vi "Find New Visa.vi"(8 "error in (no error)":errorcluster caption="entrée d'erreur (pas d'erreur)", 11 "Fonction":enum16{"Lecture Liste", "Recherche Nouveau"}(ring)=enum."Recherche Nouveau") -> (0 "error out":errorcluster caption="sortie d'erreur", 1 "Com à Initialiser":string, 2 "Trouvé":bool, 3 "liste trouvée":string[](array[string]))   [LabVIEW 2020]
uses:
  <vilib>/Instr/_visa.llb/VISA Find Search Mode.ctl
  IHM/Variable globale.vi
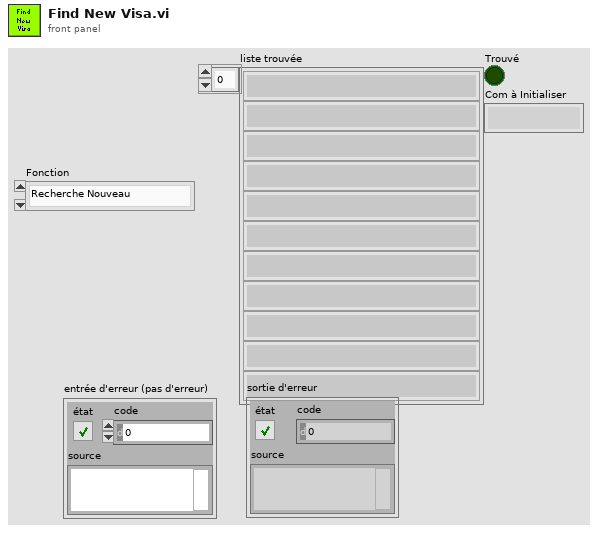
[diagram p1: front panel]
types:
  T1 = typedef "VISA Find Search Mode.ctl" = u32
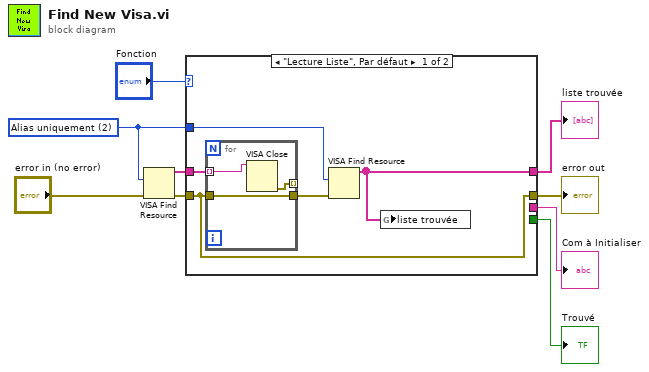
[diagram p0: block diagram]
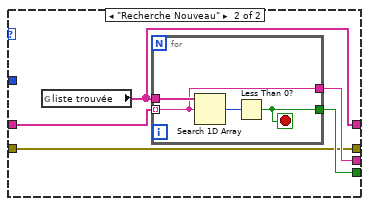
[diagram p2: hidden frame]
diagram:
  w1 = T1 2 items=["Noms canoniques uniquement"=0, "Alias uniquement"=2, "Inclure les alias correspondants"=3, "Inclure tous les alias"=4] ("Search Mode")
  n1 = VISA Find Resource(8:"error in (no error)", 10:w1) -> (0:w8:errorcluster, 3:w5:string[])  [unwired: 1 in, 1 out]
  n2 = case shown="\"Lecture Liste\", Par défaut" "Fonction" {
    tunnel: [w11 w18] -> w4
    tunnel: w5 -> [w12 w20]
    tunnel: [w14 w19] -> w2
    tunnel: w8 -> [w14 w19]
    tunnel: [_ w22] -> w7
    tunnel: [_ w21] -> w6
    tunnel: w1 -> [w10 _]
    frame "Lecture Liste", Default {
      n3 = for {
        tunnel: w12 -> [w17] mode=indexing
        tunnel: [w16] -> _ mode=indexing
        tunnel: [w15] -> w13
        tunnel: w14 -> [w15]
        n4 = VISA Close(VISA resource name=w17) -> (error out=w16:errorcluster)  [unwired: 1 in]
      }
      n5 = VISA Find Resource(8:w13, 10:w10) -> (3:w11:string[])  [unwired: 1 in, 2 out]
      n6 = global write "Variable globale.vi" "liste trouvée"(w11) -> ()
    }
    frame "Recherche Nouveau" {
      n7 = global read "Variable globale.vi" "liste trouvée"() -> (w18:string[])
      n8 = for {
        tunnel: w18 -> [w24]
        tunnel: w20 -> [w23] mode=indexing
        tunnel: [w25] -> w22
        tunnel: [w23] -> w21
        stop <- w25 stop-if-true
        n9 = Search 1D Array(1D array=w24, element=w23) -> (index of element=w26:i32)  [unwired: 1 in]
        n10 = Less Than 0?(x=w26) -> (x < 0?=w25:bool)
      }
    }
  }
  "liste trouvée" <- w4
  "Trouvé" <- w7
  "error out" <- w2
  "Com à Initialiser" <- w6
